vi "GlobalLastFrame.vi"() -> ()   [LabVIEW 2010]
panel:
  in  "Last Frame":u32
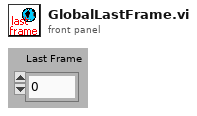
[diagram p1: front panel]
diagram:
